vi "MU Mt Analyze Result Delete.vi"(8 "error in (no error)":errorcluster, 11 "mtSynchAnalyzeResultHandle":T1) -> (0 "error out":errorcluster)   [LabVIEW 2017, in "MU_3SL_interface.lvlib"]
uses:
  MU_3SL_interface.lvlib
  handles/mtSyncAnalyzeResultHandle.ctl
  lib/MU_3SL_interface.dll
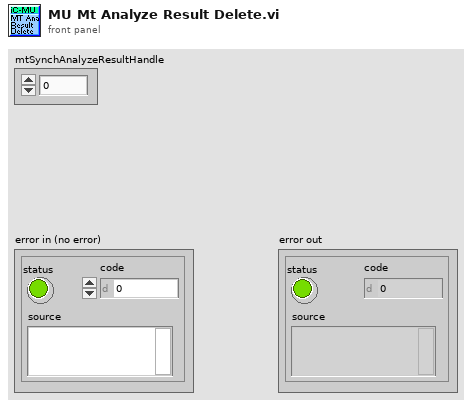
[diagram p1: front panel]
types:
  T1 = typedef "MU_3SL_interface.lvlib/mtSyncAnalyzeResultHandle.ctl" = u64
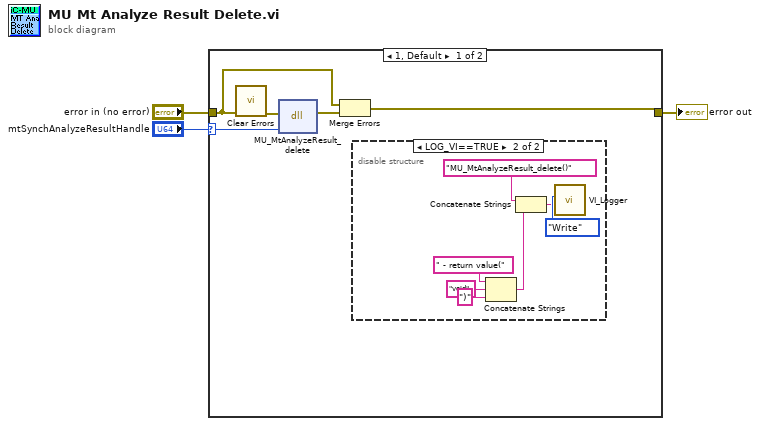
[diagram p0: block diagram]
diagram:
  n1 = case shown="1, Default" "mtSynchAnalyzeResultHandle" {
    selector: "mtSynchAnalyzeResultHandle" -> [w8 _]
    tunnel: [w4 w16] -> w3
    tunnel: "error in (no error)" -> [w5 w16]
    frame 1, Default {
      n2 = call <vilib>:"Clear Errors.vi"("error in (no error)"=w5) -> ("error out"=w7:errorcluster)  [unwired: 5 in, 1 out]
      n3 = dll-call lib="C:/Users/bes/AppData/Roaming/work/mu_9so/icsubmodules/soft_mu_3sl_master/lv_interface/lib/MU_3SL_interface**.*" fn="MU_MtAnalyzeResult_delete"(error in=w7, "mtSynchAnalyzeResultHandle"=w8) -> (error out=w6:errorcluster)  [unwired: 4 in, 1 out]
      n4 = Merge Errors(w5, w6) -> (w4:errorcluster)
      n5 = disable-structure shown="LOG_VI==TRUE" {
        frame condition #0 {
        }
        frame condition #1 (active) {
          n6 = Concatenate Strings(" - return value(" ("string"), "void" ("string"), ")" ("string")) -> (w13:string)
          n7 = Concatenate Strings("MU_MtAnalyzeResult_delete()" ("Info in"), w13) -> (w12:string)
          n8 = call "VI_Logger.vi"("Action (Read)"=enum16{"Write", "Read"}."Write", "Info in"=w12) -> ()  [unwired: 8 in, 2 out]
        }
      }
    }
    frame 0 {
    }
  }
  "error out" <- w3
